vi "Manager UI Launcher.vi"() -> ()   [LabVIEW 2021]
uses:
  363d3bde-6874-4068-849e-62e045d4c070.vi
  <vilib>/Comparison/Less/Less Functor/Less Functor.lvclass
  <vilib>/Utility/LVLibp/NI_PackedLibraryUtility.lvlib
panel:
  out "error out":errorcluster
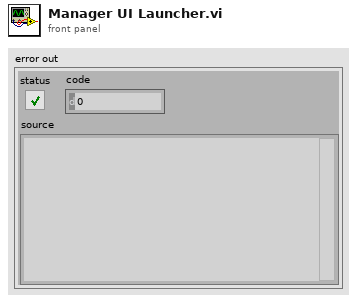
[diagram p1: front panel]
types:
  T1 = enum32{"Invalid", "Standard", "Closed", "Hidden", "Minimized", "Maximized"}
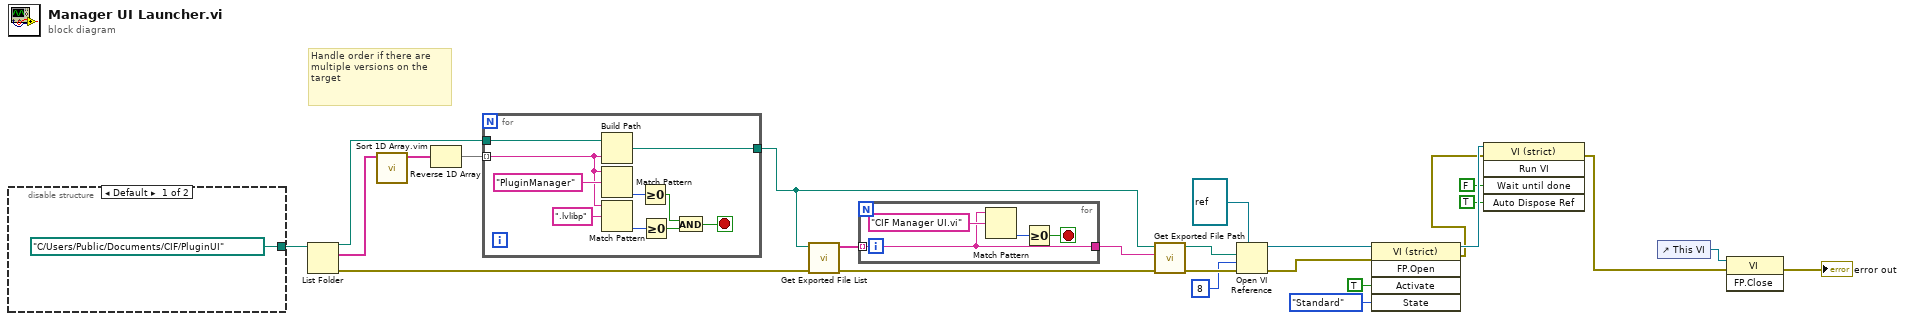
[diagram p0: block diagram]
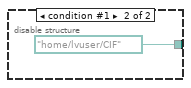
[diagram p2: hidden frame]
diagram:
  # "Handle order if there are multiple versions on the target"
  n1 = disable-structure shown="Default" {
    disable-tunnel: [path "C:/Users/Public/Documents/CIF/PluginUI" ("packed library path") path "/home/lvuser/CIF" ("packed library path")] -> w25
    frame condition #0 (active) {
    }
    frame condition #1 {
    }
  }
  n2 = List Folder(path=w25) -> (path out=w23:path, filenames=w21:string[], error out=w24:errorcluster)  [unwired: 3 in, 1 out]
  n3 = call "Sort 1D Array.vim"("unsorted array"=w21) -> ("sorted array"=w20:string[])  [unwired: 10 in]
  n4 = Reverse 1D Array(array=w20) -> (reversed array=w19:string[])
  n5 = for {
    tunnel: w19 -> [w33] mode=indexing
    tunnel: [w34] -> w22
    tunnel: w23 -> [w35]
    stop <- w28 stop-if-true
    n6 = Build Path(base path=w35, name or relative path=w33) -> (appended path=w34:path)
    n7 = Match Pattern(string=w33, regular expression="PluginManager") -> (offset past match=w37:i32)  [unwired: 1 in, 3 out]
    n8 = Match Pattern(string=w33, regular expression=".lvlibp") -> (offset past match=w31:i32)  [unwired: 1 in, 3 out]
    n9 = Greater Or Equal To 0?(x=w37) -> (x >= 0?=w29:bool)
    n10 = Greater Or Equal To 0?(x=w31) -> (x >= 0?=w30:bool)
    n11 = And(x=w29, y=w30) -> (x .and. y?=w28:bool)
  }
  n12 = call <vilib>:"Get Exported File List.vi"("error in (no error)"=w24, "packed library path"=w22) -> ("error out"=w17:errorcluster, "qualified names"=w18:string[])  [unwired: 7 in, 1 out]
  n13 = for {
    tunnel: w18 -> [w38] mode=indexing
    tunnel: [w38] -> w12
    stop <- w40 stop-if-true
    n14 = Match Pattern(string=w38, regular expression="CIF Manager UI.vi") -> (offset past match=w41:i32)  [unwired: 1 in, 3 out]
    n15 = Greater Or Equal To 0?(x=w41) -> (x >= 0?=w40:bool)
  }
  n16 = call <vilib>:"Get Exported File Path.vi"("error in (no error)"=w17, "qualified name"=w12, "packed library path"=w22) -> ("error out"=w15:errorcluster, "path"=w16:path)  [unwired: 7 in]
  n17 = Open VI Reference(type specifier VI Refnum (for type only)=refnum<vi> refnum, vi path=w16, options=8, error in (no error)=w15) -> (vi reference=w11:refnum<vi>, error out=w8:errorcluster)  [unwired: 2 in]
  n18 = invoke class="VI (strict)" method="FP.Open"(reference=w11, error in=w8, "Activate"=TRUE ("Activate?"), "State"=T1."Standard") -> (reference out=w6:refnum<vi>, error out=w3:errorcluster)  [unwired: 1 in, 3 out]
  n19 = invoke class="VI (strict)" method="Run VI"(reference=w6, error in=w3, "Wait until done"=FALSE ("Wait Until Done"), "Auto Dispose Ref"=TRUE ("Auto Dispose Reference")) -> (error out=w1:errorcluster)  [unwired: 1 in, 4 out]
  n20 = control-ref of="This VI"() -> (w2:refnum<vi>)
  n21 = invoke class="VI" method="FP.Close"(reference=w2, error in=w1) -> (error out=→"error out":errorcluster)  [unwired: 1 in, 2 out]
